vi "MonoSpec50 LargeMoveGen.vi"(4 "Abort Ref":refnum<vi>, 5 "error in":errorcluster, 6 "Moving Ref":refnum<vi>, 7 "Turns":u32=1000, 8 "Directions":bool=TRUE caption="Direction") -> (0 "error out":errorcluster, 2 "Compte":u32, 3 "timeout":bool)   [LabVIEW 2012]
doc: "Ce Vi commande la carte d'acquisition NI PCI-6052E à régler le bit de contrôle de direction et à envoyer le nombre d'impulsion voulue. Les voie de sortie utilisés pour la direction et les impulsions sont prédéterminées dans l'assistant \"Motion and Automation explorer\" (MAX)"
uses:
  <userlib>/Monospec 50/MonoSpec50 LrgMve States.ctl
  <vilib>/DAQmx/write.llb/DAQmx Write (Digital Bool 1Line 1Point).vi
  <vilib>/DAQmx/read.llb/DAQmx Read (Counter U32 1Chan 1Samp).vi
  <vilib>/DAQmx/configure/timing.llb/DAQmx Timing (Implicit).vi
  <vilib>/DAQmx/miscellaneous.llb/DAQmx Fill In Error Info.vi
  <resource>/objmgr/daqmx.rc
panel:
  out "false pulses":u32
  in  "Abort":bool
  out "Moving":bool caption="Déplacement\nen cours"
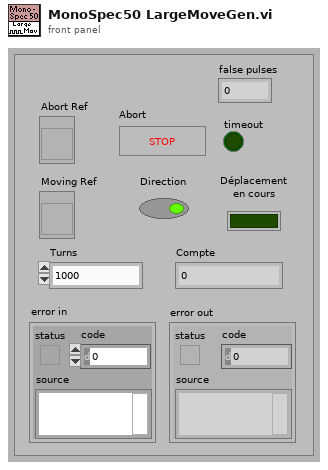
[diagram p1: front panel]
types:
  T1 = typedef "MonoSpec50 LrgMve States.ctl" = enum16{"accel2", "accel3", "decel2", "decel1", "stay1"}
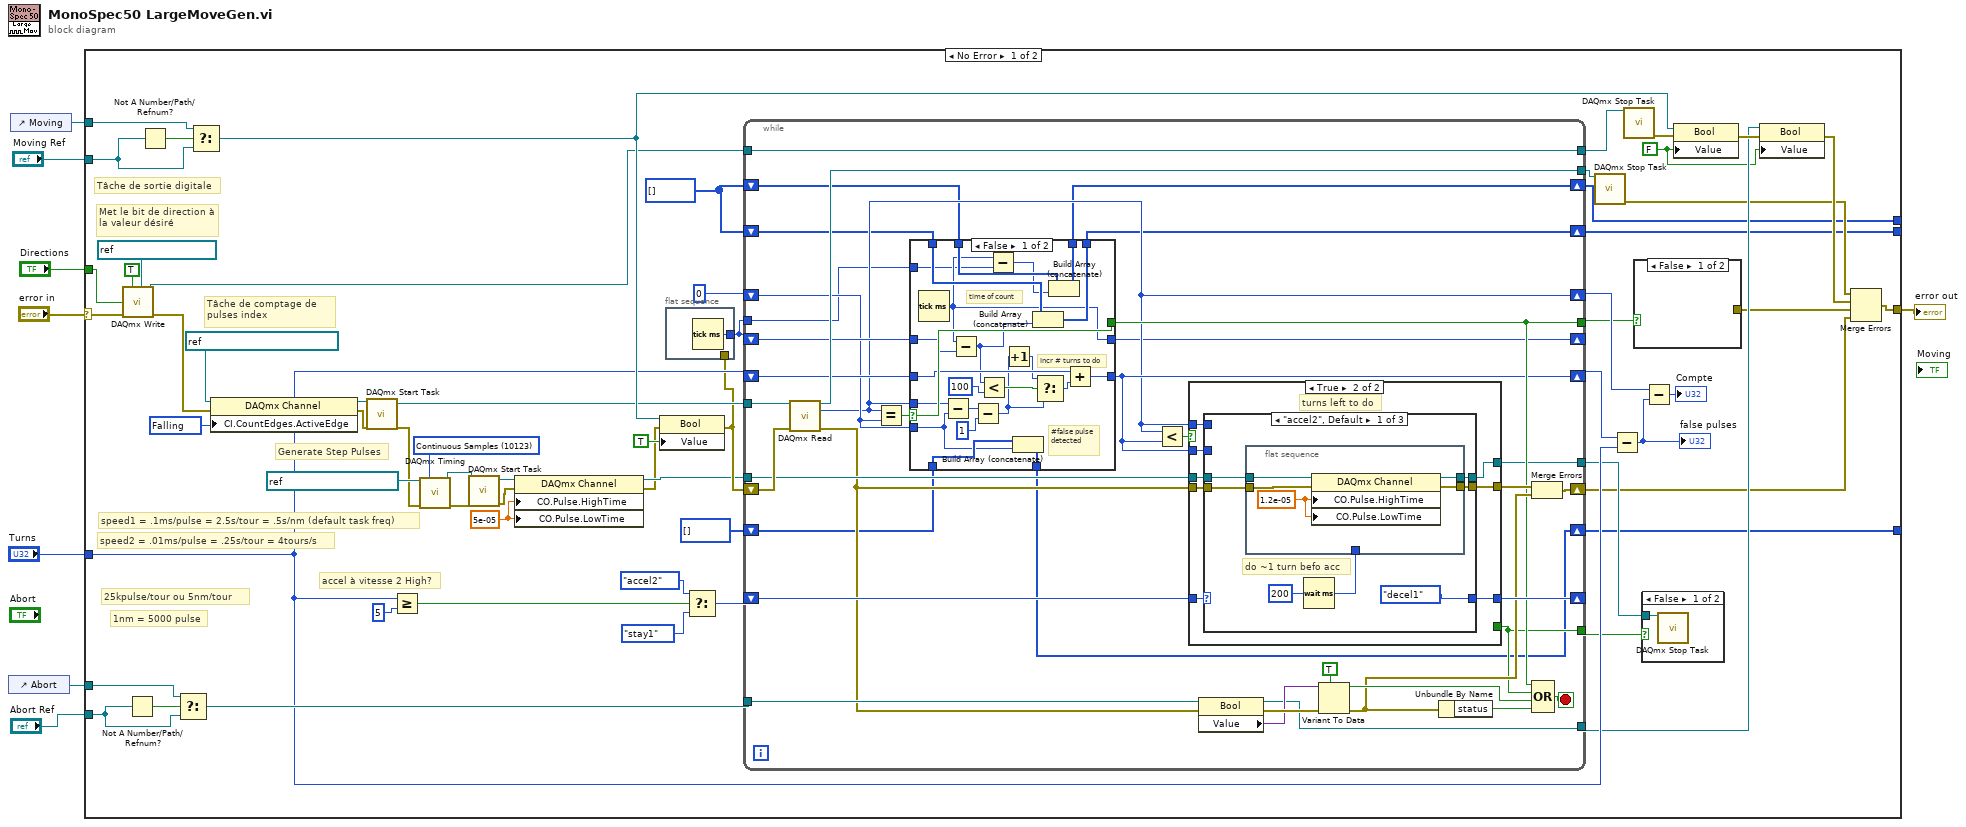
[diagram p0: block diagram]
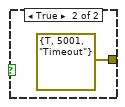
[diagram p2: hidden frame]
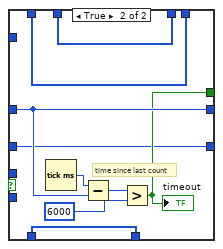
[diagram p4: hidden frame]
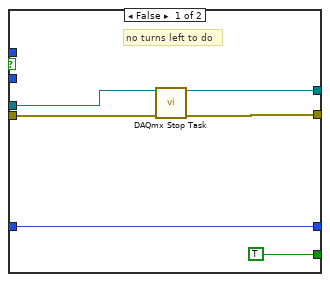
[diagram p5: hidden frame]
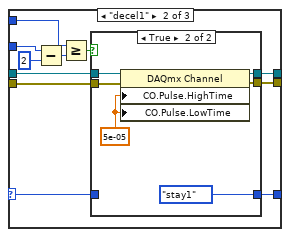
[diagram p6: hidden frame]
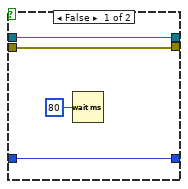
[diagram p7: hidden frame]
diagram:
  n1 = control-ref of="Abort"() -> (w2:refnum<vi>)
  n2 = control-ref of="Moving"() -> (w3:refnum<vi>)
  n3 = case shown="No Error" "error in" {
    selector: "error in" -> [w69 w193]
    tunnel: "Turns" -> [w44 _]
    tunnel: [w58 w193] -> w7
    tunnel: "Directions" -> [w50 _]
    tunnel: "Moving Ref" -> [w66 _]
    tunnel: w3 -> [w59 _]
    tunnel: w2 -> [w55 _]
    tunnel: "Abort Ref" -> [w54 _]
    tunnel: [w14 _] -> _
    tunnel: [w10 _] -> _
    tunnel: [w9 _] -> _
    frame No Error {
      w13 = u32[] []
      w17 = 10123 items=["Finite Samples"=10178, "Continuous Samples"=10123, "Hardware Timed Single Point"=12522] ("sample mode")
      w28 = 5e-05 ("CO.Pulse.HighTime")
      w39 = 10171 items=["Rising"=10280, "Falling"=10171] ("CI.CountEdges.ActiveEdge")
      w34 = FALSE ("Value")
      # "speed2 = .01ms/pulse = .25s/tour = 4tours/s"
      # "speed1 = .1ms/pulse = 2.5s/tour = .5s/nm (default task freq)"
      # "Generate Step Pulses"
      # "1nm = 5000 pulse"
      # "25kpulse/tour ou 5nm/tour"
      # "Met le bit de direction à la valeur désiré"
      # "accel à vitesse 2 High?"
      # "Tâche de comptage de pulses index"
      # "Tâche de sortie digitale"
      n4 = call-poly <vilib>:"DAQmx Write.vi"("task/channels in"=refnum<k21> "Direction Spectro", "auto start"=TRUE, "data"=w50, "error in"=w69) -> ("task out"=w20:refnum<k21>, "error out"=w48:errorcluster)  [unwired: 9 in, 1 out]
      n5 = Not A Number/Path/Refnum?(number/path/refnum=w54) -> (NaN/Path/Refnum?=w56:bool)
      n6 = Not A Number/Path/Refnum?(number/path/refnum=w66) -> (NaN/Path/Refnum?=w67:bool)
      n7 = Select(t=w55, s=w56, f=w54) -> (s? t:f=w53:refnum<vi>)
      n8 = Select(t=w59, s=w67, f=w66) -> (s? t:f=w60:refnum<vi>)
      n9 = property class="DAQmx Channel"(reference=refnum<k21> "ComptRefPulse Spectro", error in=w48, "CI.CountEdges.ActiveEdge"=w39) -> (reference out=w47:refnum<k21>, error out=w46:errorcluster)
      n10 = call <vilib>:"DAQmx Start Task.vi"("task/channels in"=w47, "error in"=w46) -> ("task out"=w45:refnum<k21>, "error out"=w15:errorcluster)  [unwired: 12 in]
      n11 = Greater Or Equal?(x=w44, y=u32 5) -> (x >= y?=w57:bool)
      n12 = call-poly <vilib>:"DAQmx Timing.vi"("task/channels in"=refnum<k21> "Sortie Pulse Spectro", "sample mode"=w17, "error in"=w15) -> ("task out"=w18:refnum<k21>, "error out"=w19:errorcluster)  [unwired: 11 in]
      n13 = call <vilib>:"DAQmx Start Task.vi"("task/channels in"=w18, "error in"=w19) -> ("task out"=w27:refnum<k21>, "error out"=w26:errorcluster)  [unwired: 12 in]
      n14 = property class="DAQmx Channel"(reference=w27, error in=w26, "CO.Pulse.HighTime"=w28, "CO.Pulse.LowTime"=w28) -> (reference out=w25:refnum<k21>, error out=w24:errorcluster)
      n15 = property class="Bool"(reference=w60, error in=w24, "Value"=TRUE) -> (error out=w29:errorcluster)  [unwired: 1 out]
      n16 = flat-sequence {
        tunnel: [w71] -> w11
        tunnel: w29 -> [_]
        frame #0 {
          n17 = Tick Count (ms)() -> (millisecond timer value=w71:u32)
        }
      }
      n18 = Select(t=MonoSpec50_LrgMve_States."accel2", s=w57, f=MonoSpec50_LrgMve_States."stay1") -> (s? t:f=w62:T1)
      n19 = while {
        tunnel: w45 -> [w110]
        tunnel: w25 -> [w97]
        shift-right: [w99] -> _
        shift-left: w62 -> [w100]
        shift-right: [w95] -> w23
        shift-left: w29 -> [w109]
        tunnel: w53 -> [w104]
        tunnel: [w98] -> w52
        shift-right: [w84] -> w41
        shift-left: u32 0 -> [w85]
        shift-right: [w81] -> _
        shift-left: w11 -> [w91]
        tunnel: [w90] -> w31
        shift-right: [w88] -> w43
        shift-left: w44 -> [w89]
        tunnel: [w87] -> w32
        tunnel: [w86] -> w33
        tunnel: [w83] -> w37
        tunnel: [w82] -> w21
        tunnel: w20 -> [w82]
        shift-right: [w79] -> w14
        shift-left: w13 -> [w80]
        shift-right: [w76] -> w9
        shift-left: w13 -> [w77]
        shift-right: [w74] -> w10
        shift-left: u32[] [] -> [w78]
        tunnel: w11 -> [w75]
        stop <- w108 stop-if-true
        n20 = call-poly <vilib>:"DAQmx Read.vi"("task/channels in"=w110, "error in"=w109) -> ("task out"=w98:refnum<k21>, "data"=w84:u32, "error out"=w96:errorcluster)  [unwired: 11 in]
        n21 = Equal?(x=w84, y=w85) -> (x = y?=w92:bool)
        n22 = case shown="False" w92 {
          selector: w92 -> [w133 _]
          tunnel: w91 -> [w127 w139]
          tunnel: [w122 w139] -> w81
          tunnel: w85 -> [w118 _]
          tunnel: [w133 w138] -> w90
          tunnel: w84 -> [w129 _]
          tunnel: w89 -> [w128 w137]
          tunnel: [w130 w137] -> w88
          tunnel: w80 -> [w126 w136]
          tunnel: [w125 w136] -> w79
          tunnel: w78 -> [w119 w134]
          tunnel: w77 -> [w124 w135]
          tunnel: [w123 w135] -> w76
          tunnel: w75 -> [w121 _]
          tunnel: [w117 w134] -> w74
          frame False {
            # "time of count"
            # "Incr # turns to do"
            # "#false pulse\ndetected"
            n23 = Tick Count (ms)() -> (millisecond timer value=w122:u32)
            n24 = Subtract(x=w129, y=w118) -> (x-y=w132:u32)
            n25 = Subtract(x=w122, y=w127) -> (x-y=w116:u32)
            n26 = Subtract(x=w132, y=u32 1) -> (x-y=w113:u32)
            n27 = Less?(x=w116, y=u32 100) -> (x < y?=w115:bool)
            n28 = Subtract(x=w122, y=w121) -> (x-y=w120:u32)
            n29 = Increment(x=w113) -> (x+1=w111:u32)
            n30 = Build Array (concatenate)(w119, w118) -> (w117:u32[])
            n31 = Build Array (concatenate)(w126, w116) -> (w125:u32[])
            n32 = Select(t=w111, s=w115, f=w113) -> (s? t:f=w114:u32)
            n33 = Build Array (concatenate)(w124, w120) -> (w123:u32[])
            n34 = Add(x=w128, y=w114) -> (x+y=w130:u32)
          }
          frame True {
            # "time since last count"
            n35 = Tick Count (ms)() -> (millisecond timer value=w140:u32)
            n36 = Subtract(x=w140, y=w139) -> (x-y=w142:u32)
            n37 = Greater?(x=w142, y=u32 6000) -> (0:w138:bool)
            "timeout" <- w138
          }
        }
        n38 = Less?(x=w84, y=w88) -> (x < y?=w103:bool)
        n39 = case shown="True" w103 {
          tunnel: [TRUE ("Value") _] -> w87
          tunnel: w100 -> [w147 w156]
          tunnel: [w147 w155] -> w99
          tunnel: w97 -> [w146 w154]
          tunnel: w96 -> [w145 w153]
          tunnel: [w144 w152] -> w93
          tunnel: w84 -> [_ w151]
          tunnel: w88 -> [_ w150]
          tunnel: [w143 w149] -> w86
          frame False {
            # "no turns left to do"
            n40 = call <vilib>:"DAQmx Stop Task.vi"("task/channels in"=w146, "error in"=w145) -> ("task out"=w143:refnum<k21>, "error out"=w144:errorcluster)  [unwired: 12 in]
          }
          frame True {
            # "turns left to do"
            n41 = case shown="\"accel2\", Default" w156 {
              selector: w156 -> [_ w173 w192]
              tunnel: [MonoSpec50_LrgMve_States."decel1" w172 w192] -> w155
              tunnel: w154 -> [w163 w179 w191]
              tunnel: w153 -> [w162 w178 w190]
              tunnel: [w161 w176 w190] -> w152
              tunnel: w151 -> [_ w175 _]
              tunnel: [w159 w177 w191] -> w149
              tunnel: w150 -> [_ w170 _]
              frame "accel2", Default {
                # "do ~1 turn befo acc"
                n42 = flat-sequence {
                  tunnel: w163 -> [w168]
                  tunnel: w162 -> [w167]
                  tunnel: [w165] -> w161
                  tunnel: [w164] -> w159
                  tunnel: w157 -> [_]
                  frame #0 {
                    w166 = 1.2e-05 ("CO.Pulse.HighTime")
                    n43 = property class="DAQmx Channel"(reference=w168, error in=w167, "CO.Pulse.HighTime"=w166, "CO.Pulse.LowTime"=w166) -> (reference out=w164:refnum<k21>, error out=w165:errorcluster)
                  }
                }
                n44 = Wait (ms)(milliseconds to wait=u32 200) -> (millisecond timer value=w157:u32)
              }
              frame "decel1" {
                n45 = Subtract(x=w170, y=u32 2) -> (x-y=w169:u32)
                n46 = Greater Or Equal?(x=w175, y=w169) -> (x >= y?=w174:bool)
                n47 = case shown="True" w174 {
                  tunnel: w179 -> [w183 w189]
                  tunnel: w178 -> [w182 w188]
                  tunnel: [w183 w187] -> w177
                  tunnel: [w182 w186] -> w176
                  tunnel: w173 -> [w180 _]
                  tunnel: [w180 MonoSpec50_LrgMve_States."stay1"] -> w172
                  frame False {
                    n48 = Wait (ms)(milliseconds to wait=u32 80) -> ()  [unwired: 1 out]
                  }
                  frame True {
                    w185 = 5e-05 ("CO.Pulse.HighTime")
                    n49 = property class="DAQmx Channel"(reference=w189, error in=w188, "CO.Pulse.HighTime"=w185, "CO.Pulse.LowTime"=w185) -> (reference out=w187:refnum<k21>, error out=w186:errorcluster)
                  }
                }
              }
              frame "stay1" {
              }
            }
          }
        }
        n50 = property class="Bool"(reference=w104, error in=w96) -> (reference out=w83:refnum<vi>, error out=w107:errorcluster, "Value"=w106:variant)
        n51 = Variant To Data(error in=w107, type=TRUE ("Value"), Variant=w106) -> (data=w101:bool, error out=w94:errorcluster)
        n52 = Unbundle By Name(w94) -> ("status"=w102:bool)
        n53 = Merge Errors(w93, w94) -> (w95:errorcluster)
        n54 = Compound Arithmetic op=OR(w90, w87, w101, w102) -> (w108:bool)
      }
      n55 = call <vilib>:"DAQmx Stop Task.vi"("task/channels in"=w52) -> ("error out"=w22:errorcluster)  [unwired: 13 in, 1 out]
      n56 = Subtract(x=w43, y=w44) -> (x-y=w42:u32)
      "false pulses" <- w42
      n57 = call <vilib>:"DAQmx Stop Task.vi"("task/channels in"=w21) -> ("error out"=w35:errorcluster)  [unwired: 13 in, 1 out]
      n58 = case shown="False" w31 {
        tunnel: [_ errorcluster {"status"=TRUE, "code"=5001, "source"="Timeout"} ("error constant")] -> w30
        frame False {
        }
        frame True {
        }
      }
      n59 = case shown="False" w32 {
        tunnel: w33 -> [w73 _]
        frame False {
          n60 = call <vilib>:"DAQmx Stop Task.vi"("task/channels in"=w73) -> ()  [unwired: 13 in, 2 out]
        }
        frame True {
        }
      }
      n61 = Subtract(x=w41, y=w42) -> (x-y=→"Compte":u32)
      n62 = property class="Bool"(reference=w60, error in=w35, "Value"=w34) -> (error out=w38:errorcluster)  [unwired: 1 out]
      n63 = property class="Bool"(reference=w37, error in=w38, "Value"=w34) -> (error out=w36:errorcluster)  [unwired: 1 out]
      n64 = Merge Errors(w22, w36, w30, w23) -> (w58:errorcluster)
    }
    frame Error {
    }
  }
  "error out" <- w7
